vi "ke37xx Get Closed List.vi"(0 "VISA Resource Name":refnum<visa-resource-name>, 1 "Channel List":string, 11 "error in (no error)":errorcluster, 12 "Bytes To Read (1024)":u32=1024) -> (4 "VISA Resource Name Out":refnum<visa-resource-name>, 8 "Closed List":string, 15 "error out":errorcluster)   [LabVIEW 2009, in "Keithley 3700 Series.lvlib"]
doc: "This VI allows you to set, query, or clear the list of channels that are forbidden to be closed."
uses:
  <instrlib>/Keithley 3706/Keithley 3700 Series.lvlib
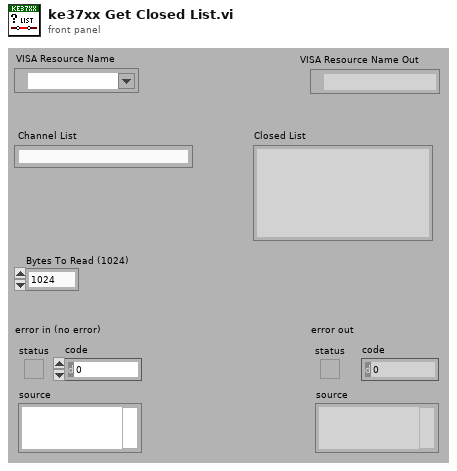
[diagram p1: front panel]
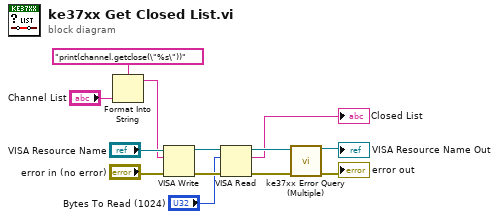
[diagram p0: block diagram]
diagram:
  n1 = Format Into String(format string="print(channel.getclose(\"%s\"))", "Channel List") -> (resulting string=w1:string)  [unwired: 2 in, 1 out]
  n2 = VISA Write(VISA resource name="VISA Resource Name", write buffer=w1, error in (no error)="error in (no error)") -> (VISA resource name out=w5:refnum<visa-resource-name>, error out=w4:errorcluster)  [unwired: 1 out]
  n3 = VISA Read(VISA resource name=w5, byte count="Bytes To Read (1024)", error in (no error)=w4) -> (VISA resource name out=w9:refnum<visa-resource-name>, read buffer=→"Closed List":string, error out=w8:errorcluster)  [unwired: 1 out]
  n4 = call <instrlib>:"ke37xx Error Query (Multiple).vi"("VISA resource name"=w9, "error in (no error)"=w8) -> ("VISA resource name out"=→"VISA Resource Name Out":refnum<visa-resource-name>, "error out"=→"error out":errorcluster)  [unwired: 12 out]
